vi "RTS Macro Calc Cycle Times.vi"(0 "Time":dbl[](array[numeric]) format="%<%H:%M:%S>t", 5 "Refrigeration Core Stats Input":T1 {"Average Compressor Cycle Time (Min)" format="%0.2f"; "Average Compressor Power (W)" format="%0.2f"; "Power Start Time (sec)" format="%<%H:%M:%S>t"; "Power End time (sec)" format="%<%H:%M:%S>t"; "Average Defrost Power (W)" format="%0.2f"}, 11 "Error In":errorcluster, 12 "Filtered Pulse Train":dbl[](array[numeric])=array[53894 elements]) -> (3 "Defrost/Cycle Times":dbl[](array[numeric]), 6 "Refrigeration Core Stats Output":T1 {"Average Compressor Cycle Time (Min)" format="%0.2f"; "Average Compressor Power (W)" format="%0.2f"; "Power Start Time (sec)" format="%<%H:%M:%S>t"; "Power End time (sec)" format="%<%H:%M:%S>t"; "Average Defrost Power (W)" format="%0.2f"}, 13 "Time @ Index":dbl[](array[numeric]) format="%<%H:%M:%S>t", 14 "Transistion Index Locations":i32[](array[numeric]), 15 "Error Out":errorcluster)   [LabVIEW 2016]
uses:
  Type Definitions/RTS Macro Refrigeration Core Stats.ctl
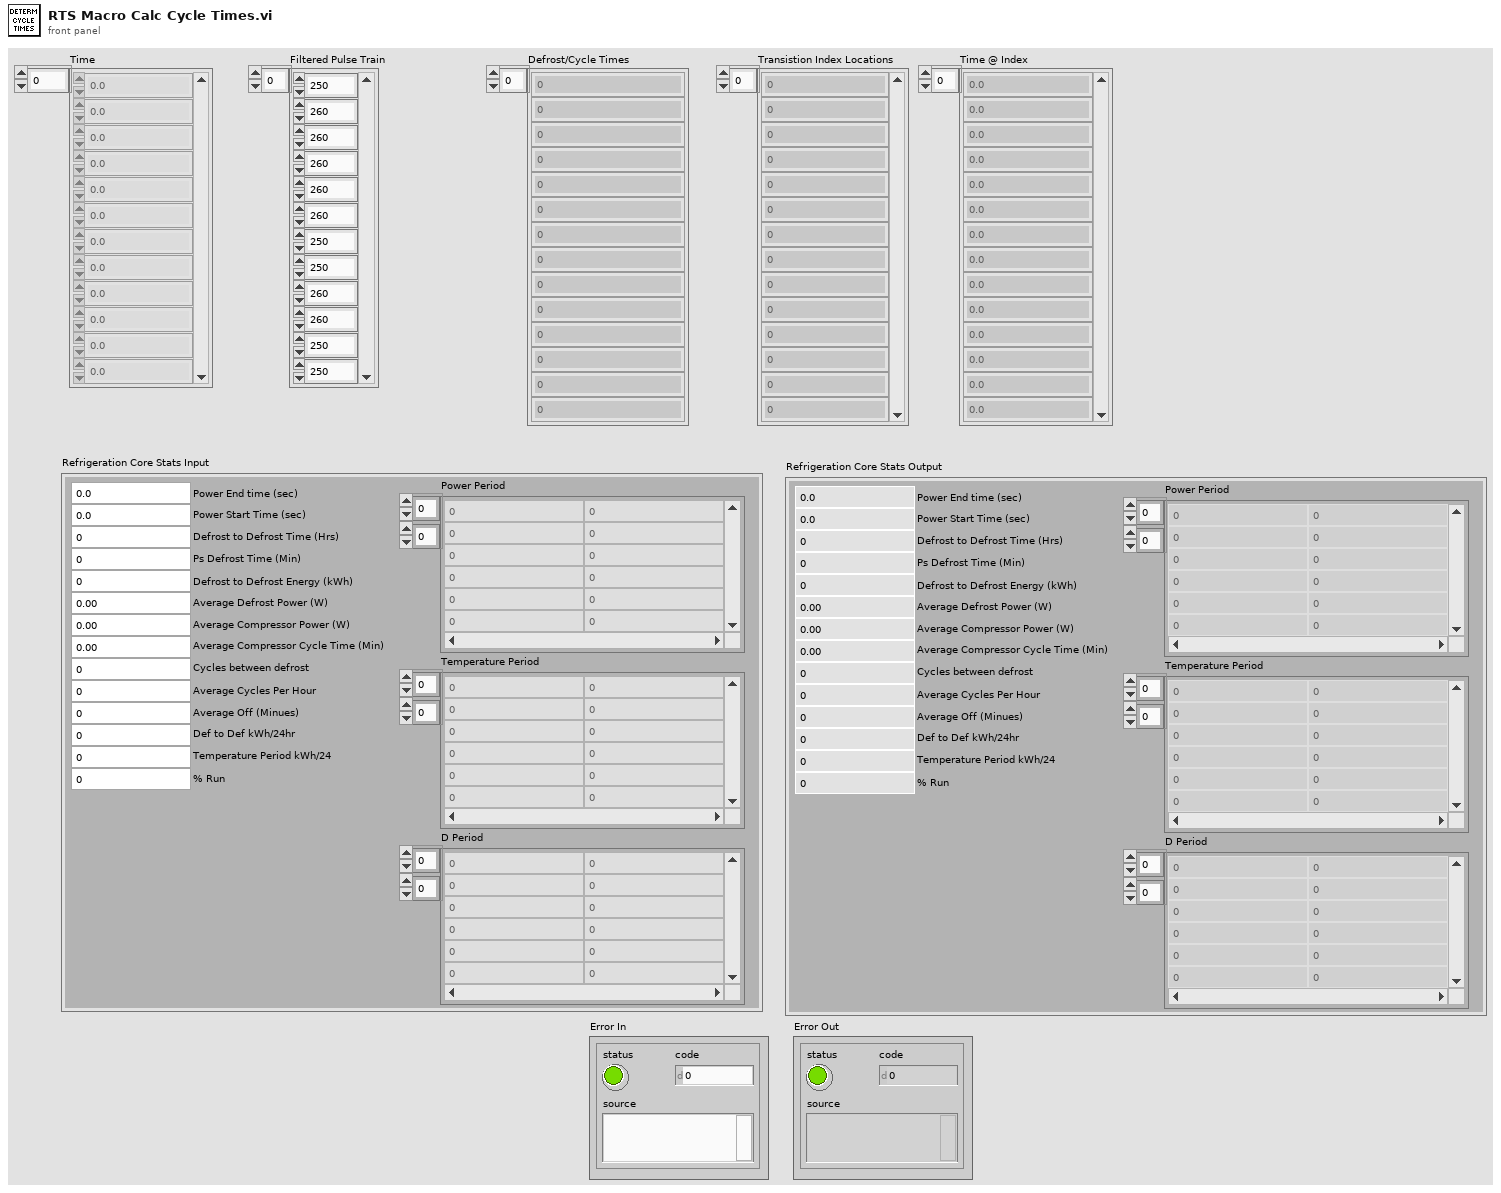
[diagram p1: front panel]
types:
  T1 = typedef "RTS Macro Refrigeration Core Stats.ctl" = cluster{"Average Defrost Power (W)":dbl, "Power End time (sec)":dbl, "Power Start Time (sec)":dbl, "Defrost to Defrost Time (Hrs)":dbl, "Ps Defrost Time (Min)":dbl, "Defrost to Defrost Energy (kWh)":dbl, "Average Compressor Power (W)":dbl, "Average Compressor Cycle Time (Min)":dbl, "Power Period":dbl[][], "Cycles between defrost":i32, "Average Cycles Per Hour":dbl, "Average Off (Minues)":dbl, "Def to Def kWh/24hr":dbl, "Temperature Period kWh/24":dbl, "% Run":dbl, "Temperature Period":dbl[][], "D Period":dbl[][]}
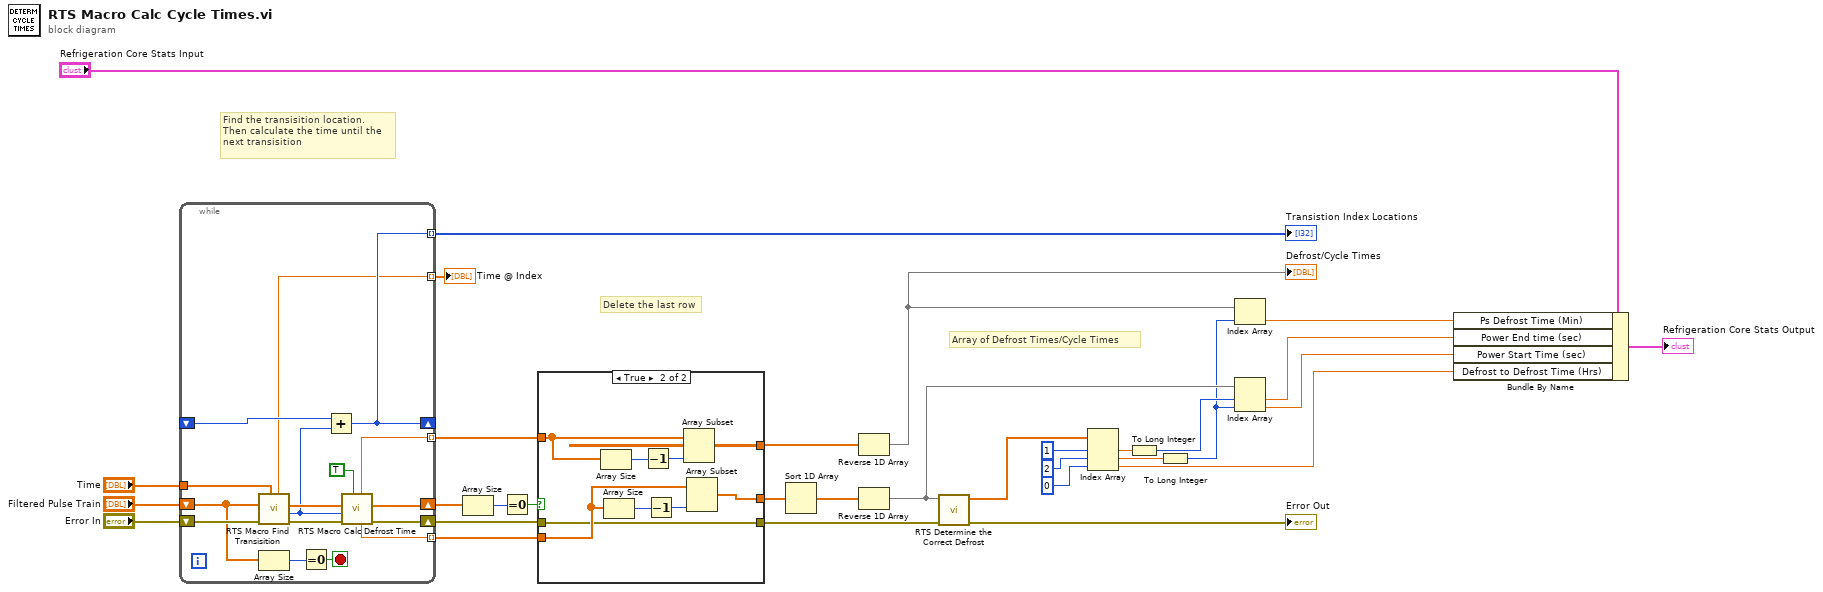
[diagram p0: block diagram]
diagram:
  # "Array of Defrost Times/Cycle Times"
  # "Delete the last row"
  # "Find the transisition location.\nThen calculate the time until the\nnext transisition"
  n1 = while {
    shift-right: [w44] -> w30
    shift-left: "Filtered Pulse Train" -> [w42]
    shift-right: [w46] -> w14
    shift-left: "Error In" -> [w47]
    tunnel: [w45] -> w29 mode=indexing
    tunnel: [w39] -> w28 mode=indexing
    shift-right: [w36] -> _
    shift-left: _ -> [w37]
    tunnel: [w36] -> w10 mode=indexing
    tunnel: [w34] -> w3 mode=indexing
    tunnel: "Time" -> [w33]
    stop <- w40 stop-if-true
    n2 = call "RTS Macro Find Transisition.vi"("Time"=w33, "Error In"=w47, "Input Pulse Train"=w42) -> ("Error Out"=w48:errorcluster, "Transisition Index"=w38:i32, "Output Dataset"=w43:dbl[], "Transistion Timestamp"=w34:dbl)  [unwired: 5 in]
    n3 = Array Size(array=w42) -> (size(s)=w41:i32)
    n4 = Equal To 0?(x=w41) -> (x = 0?=w40:bool)
    n5 = Add(x=w37, y=w38) -> (x+y=w36:i32)
    n6 = call "RTS Macro Calc Defrost Time.vi"("Use Filter?"=TRUE, "Error In"=w48, "Transisition Index"=w38, "Input Data"=w43) -> ("Error Out"=w46:errorcluster, "Parsed Output Data"=w44:dbl[], "min value"=w39:dbl, "Defrost Time (Min)"=w45:dbl)  [unwired: 3 in, 1 out]
  }
  "Transistion Index Locations" <- w10
  "Time @ Index" <- w3
  n7 = Array Size(array=w30) -> (size(s)=w32:i32)
  n8 = Equal To 0?(x=w32) -> (x = 0?=w31:bool)
  n9 = case shown="True" w31 {
    tunnel: w29 -> [w51 w59]
    tunnel: [w51 w60] -> w17
    tunnel: w28 -> [w50 w53]
    tunnel: [w50 w54] -> w27
    tunnel: w14 -> [w49 w52]
    tunnel: [w49 w52] -> w13
    frame False {
    }
    frame True {
      n10 = Array Size(array=w59) -> (size(s)=w58:i32)
      n11 = Array Size(array=w53) -> (size(s)=w55:i32)
      n12 = Decrement(x=w58) -> (x-1=w57:i32)
      n13 = Decrement(x=w55) -> (x-1=w56:i32)
      n14 = Array Subset(array=w59, length=w57) -> (w60:dbl[])  [unwired: 1 in]
      n15 = Array Subset(array=w53, length=w56) -> (w54:dbl[])  [unwired: 1 in]
    }
  }
  n16 = Sort 1D Array(array=w27) -> (sorted array=w26:dbl[])
  n17 = Reverse 1D Array(array=w17) -> (reversed array=w11:dbl[])
  "Defrost/Cycle Times" <- w11
  n18 = Reverse 1D Array(array=w26) -> (reversed array=w22:dbl[])
  n19 = call "RTS Determine the Correct Defrost.vi"("Error In"=w13, "Defrost Info Input"=w22) -> ("Error Out"=→"Error Out":errorcluster, "Longest Defrost Cycle data"=w25:dbl[])  [unwired: 8 in]
  n20 = Index Array(array=w25, index #1=1 ("index"), index #2=2 ("index"), index #3=0 ("index")) -> (element #1=w21:dbl, element #2=w20:dbl, element #3=w5:dbl)
  n21 = To Long Integer(number=w21) -> (32bit integer=w19:i32)
  n22 = To Long Integer(number=w20) -> (32bit integer=w16:i32)
  n23 = Index Array(array=w11, index=w16) -> (element=w8:dbl)
  n24 = Index Array(array=w22, index #1=w19, index #2=w16) -> (element #1=w7:dbl, element #2=w6:dbl)
  n25 = Bundle By Name(cluster="Refrigeration Core Stats Input", "Ps Defrost Time (Min)"=w8, "Power End time (sec)"=w7, "Power Start Time (sec)"=w6, "Defrost to Defrost Time (Hrs)"=w5) -> (→"Refrigeration Core Stats Output":T1)
